vi "ReadAppKeyFile.vi"(7 "Task":enum16{"Read", "Write"}(ring), 8 "error in (no error)":errorcluster, 11 "Device In":T1={"Name"="", "BaseURL"="", "AppKey"="", "Headers"=["Content-Type:application/json"], "Timeout"=10000}) -> (0 "error out":errorcluster, 2 "text":string, 3 "Device Out":T1={"Name"="", "BaseURL"="", "AppKey"="", "Headers"=["Content-Type:application/json"], "Timeout"=10000})   [LabVIEW 2019]
uses:
  <userlib>/MicroPython/VIs/SystemLink/SkylineCluster.ctl
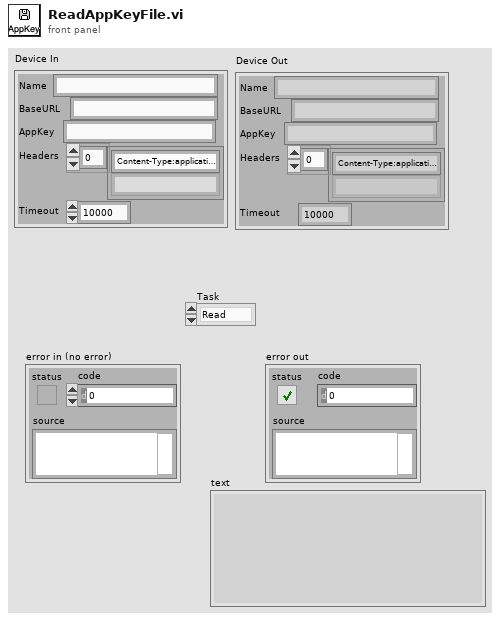
[diagram p1: front panel]
types:
  T1 = cluster{"Name":string, "BaseURL":string, "AppKey":string, "Headers":string[], "Timeout":i32}
  T2 = typedef "SkylineCluster.ctl" = cluster{"Name":string, "BaseURL":string, "AppKey":string, "Headers":string[], "Timeout":i32}
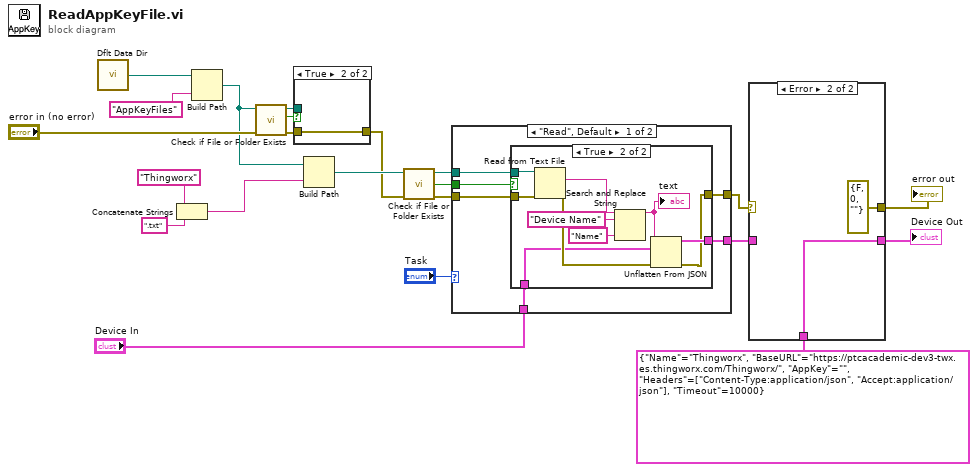
[diagram p0: block diagram]
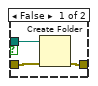
[diagram p2: hidden frame]
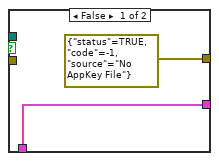
[diagram p4: hidden frame]
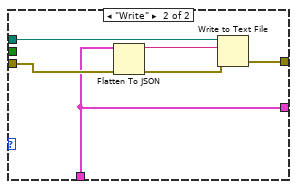
[diagram p5: hidden frame]
diagram:
  n1 = call <vilib>:"Dflt Data Dir.vi"() -> ("App:Default Data Directory"=w8:path)
  n2 = Concatenate Strings("Thingworx" ("Name"), ".txt" ("string")) -> (w21:string)
  n3 = Build Path(base path=w8, name or relative path="AppKeyFiles") -> (appended path=w4:path)
  n4 = call <vilib>:"Check if File or Folder Exists.vi"("error in (no error)"="error in (no error)", "path"=w4) -> ("error out"=w5:errorcluster, "file or folder exists?"=w7:bool, "dup path"=w6:path)  [unwired: 7 in]
  n5 = case shown="True" w7 {
    tunnel: w6 -> [w25 _]
    tunnel: w5 -> [w24 w26]
    tunnel: [w23 w26] -> w13
    frame False {
      n6 = Create Folder(path (use dialog)=w25, error in=w24) -> (error out=w23:errorcluster)  [unwired: 1 in, 2 out]
    }
    frame True {
    }
  }
  n7 = Build Path(base path=w4, name or relative path=w21) -> (appended path=w20:path)
  n8 = call <vilib>:"Check if File or Folder Exists.vi"("error in (no error)"=w13, "path"=w20) -> ("error out"=w18:errorcluster, "file or folder exists?"=w16:bool, "dup path"=w19:path)  [unwired: 7 in]
  n9 = case shown="\"Read\", Default" "Task" {
    tunnel: w19 -> [w31 w50]
    tunnel: w18 -> [w32 w48]
    tunnel: [w30 w46] -> w12
    tunnel: w16 -> [w29 _]
    tunnel: [w28 w45] -> w11
    tunnel: "Device In" -> [w27 w45]
    frame "Read", Default {
      n10 = case shown="True" w29 {
        tunnel: w32 -> [_ w44]
        tunnel: w31 -> [_ w43]
        tunnel: [errorcluster {"status"=TRUE, "code"=-1, "source"="No AppKey File"} ("error out") w39] -> w30
        tunnel: [w33 w40] -> w28
        tunnel: w27 -> [w33 w41]
        frame False {
        }
        frame True {
          n11 = Read from Text File(file (use dialog)=w43, error in=w44) -> (text=w38:string, error out=w42:errorcluster)  [unwired: 2 in, 2 out]
          n12 = Search and Replace String(input string=w38, search string="Device Name", replace string="Name" ("replace string (\"\")")) -> (result string=w35:string)  [unwired: 5 in, 3 out]
          "text" <- w35
          n13 = Unflatten From JSON(JSON string=w35, type and defaults=w41, error in (no error)=w42) -> (value=w40:T1, error out=w39:errorcluster)  [unwired: 4 in]
        }
      }
    }
    frame "Write" {
      n14 = Flatten To JSON(anything=w45, error in (no error)=w48) -> (JSON string=w49:string, 11:w47:errorcluster)  [unwired: 1 in]
      n15 = Write to Text File(file (use dialog)=w50, text=w49, error in=w47) -> (error out=w46:errorcluster)  [unwired: 1 in, 2 out]
    }
  }
  n16 = case shown="Error" w12 {
    selector: w12 -> [w51 _]
    tunnel: [w52 w53] -> w1
    tunnel: w11 -> [w52 _]
    tunnel: [w51 errorcluster {"status"=FALSE, "code"=0, "source"=""} ("error IO")] -> w10
    tunnel: T2 {"Name"="Thingworx", "BaseURL"="https://ptcacademic-dev3-twx.es.thingworx.com/Thingworx/", "AppKey"="", "Headers"=["Content-Type:application/json", "Accept:application/json"], "Timeout"=10000} ("Device In") -> [_ w53]
    frame No Error {
    }
    frame Error {
    }
  }
  "error out" <- w10
  "Device Out" <- w1
